vi "Lab3LabVIEW.vi"() -> ()   [LabVIEW 2019]
uses:
  <vilib>/Instr/_visa.llb/VISA Configure Serial Port (Instr).vi
  <vilib>/Utility/file.llb/Write Delimited Spreadsheet (DBL).vi
panel:
  out "Moisture Index":dbl
  out "Moisture Collection":dbl(graph)
  out "array w/ subset deleted":dbl[][](array[numeric])
  out "Wet":bool
  out "Flooded":bool
  out "Drought":bool
  in  "?":bool
  in  "Arduino COM Port":refnum<visa-resource-name>="COM3"
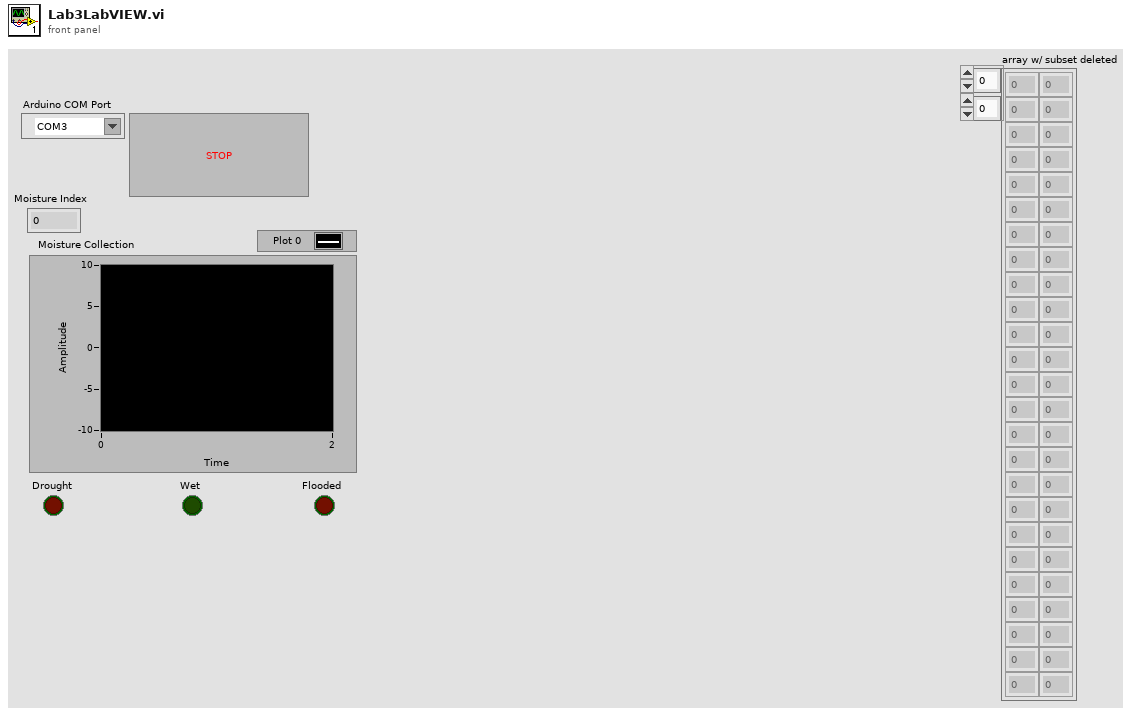
[diagram p1: front panel]
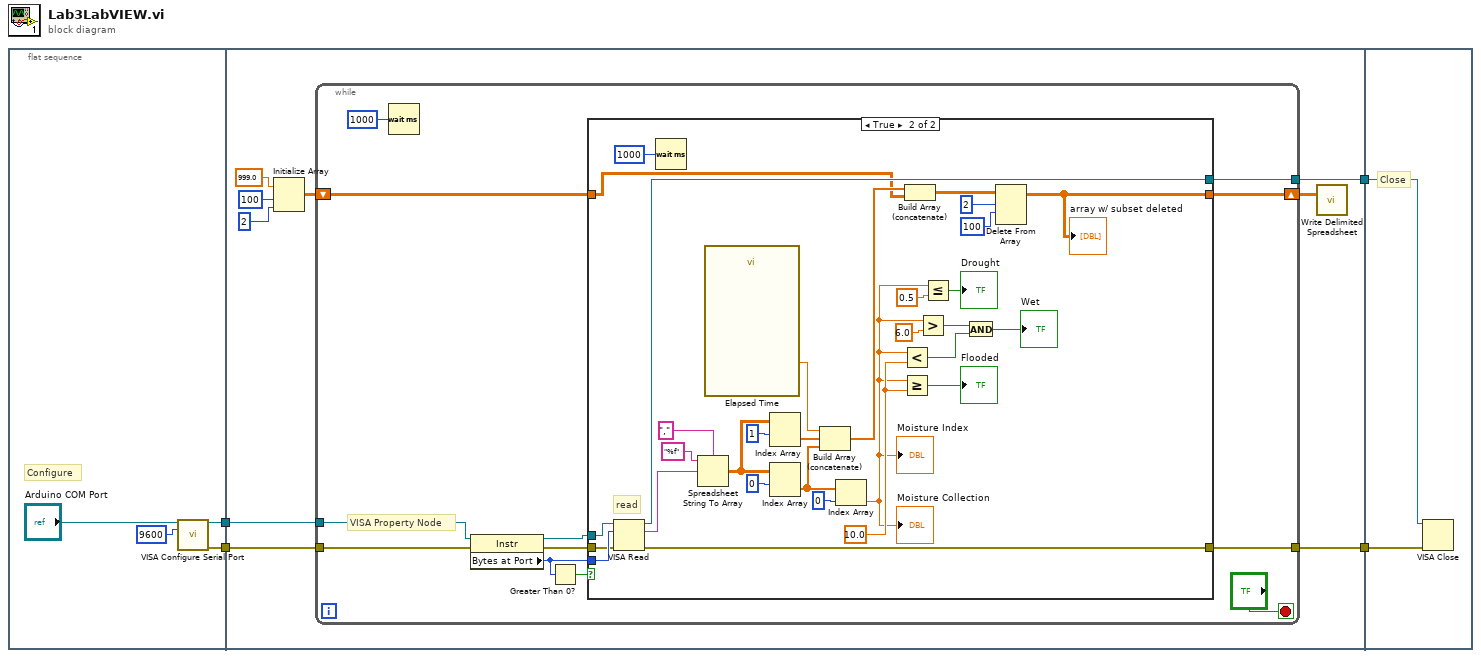
[diagram p0: block diagram]
diagram:
  n1 = flat-sequence {
    tunnel: [w6] -> w4
    tunnel: [w5] -> w3
    tunnel: w4 -> [w17]
    tunnel: [w16] -> w2
    tunnel: w3 -> [w15]
    tunnel: [w14] -> w1
    tunnel: w2 -> [w65]
    tunnel: w1 -> [w64]
    frame #0 {
      # "Configure"
      n2 = call-poly "VISA Configure Serial Port"("VISA resource name"="Arduino COM Port", "baud rate (9600)"=u32 9600) -> ("VISA resource name out"=w6:refnum<visa-resource-name>, "error out"=w5:errorcluster)  [unwired: 12 in]
    }
    frame #1 {
      n3 = Initialize Array(999.0 ("element"), 100 ("dimension size"), 2 ("dimension size")) -> (w10:dbl[][])
      n4 = while {
        tunnel: w17 -> [w21]
        tunnel: [w24] -> w16
        tunnel: w15 -> [w20]
        tunnel: [w22] -> w14
        shift-right: [w18] -> w9
        shift-left: w10 -> [w19]
        stop <- "?" stop-if-true
        # "VISA Property Node"
        n5 = Wait (ms)(milliseconds to wait=u32 1000) -> ()  [unwired: 1 out]
        n6 = property class="Instr"(reference=w21, error in=w20) -> (reference out=w28:refnum<visa-resource-name>, error out=w23:errorcluster, "Bytes at Port"=w27:u32)
        n7 = Greater Than 0?(x=w27) -> (x > 0?=w29:bool)
        n8 = case shown="True" w29 {
          tunnel: w28 -> [w32 w63]
          tunnel: [w32 w62] -> w24
          tunnel: w27 -> [_ w58]
          tunnel: w23 -> [w31 w57]
          tunnel: [w31 w56] -> w22
          tunnel: w19 -> [w30 w49]
          tunnel: [w30 w45] -> w18
          frame False {
          }
          frame True {
            w36 = 10.0 ("y")
            # "read"
            n9 = VISA Read(VISA resource name=w63, byte count=w58, error in (no error)=w57) -> (VISA resource name out=w62:refnum<visa-resource-name>, read buffer=w61:string, error out=w56:errorcluster)  [unwired: 1 out]
            n10 = Wait (ms)(milliseconds to wait=u32 1000) -> ()  [unwired: 1 out]
            n11 = Spreadsheet String To Array(delimiter (Tab)=",", format string="%f", spreadsheet string=w61) -> (array=w39:dbl[][])  [unwired: 1 in]
            n12 = call "Elapsed Time"() -> ("Elapsed Time (s)"=w52:dbl)  [unwired: 12 in, 7 out]
            n13 = Index Array(array=w39, index (row)=1) -> (element=w51:dbl[])  [unwired: 1 in]
            n14 = Index Array(array=w39, index (row)=0) -> (element=w35:dbl[])  [unwired: 1 in]
            n15 = Build Array (concatenate)(w52, w51, w35) -> (w50:dbl[])
            n16 = Index Array(array=w35, index=0) -> (element=w33:dbl)
            "Moisture Collection" <- w33
            "Moisture Index" <- w33
            n17 = Less?(x=w33, y=w36) -> (x < y?=w41:bool)
            n18 = Greater Or Equal?(x=w33, y=w36) -> (x >= y?=→"Flooded":bool)
            n19 = Build Array (concatenate)(w50, w49) -> (w48:dbl[][])
            n20 = Greater?(x=w33, y=6.0) -> (0:w43:bool)
            n21 = Less Or Equal?(x=w33, y=0.5) -> (x <= y?=→"Drought":bool)
            n22 = And(x=w43, y=w41) -> (x .and. y?=→"Wet":bool)
            n23 = Delete From Array(array=w48, length=2, index (row)=100) -> (array with subset deleted=w45:dbl[][])  [unwired: 1 in, 1 out]
            "array w/ subset deleted" <- w45
          }
        }
      }
      n24 = call-poly <vilib>:"Write Delimited Spreadsheet.vi"("2D data"=w9) -> ()  [unwired: 13 in, 2 out]
    }
    frame #2 {
      # "Close"
      n25 = VISA Close(VISA resource name=w65, error in (no error)=w64) -> ()  [unwired: 1 out]
    }
  }
